vi "DeQueue State.vi"(8 "error in":errorcluster, 10 "Timeout (-1)":i32=-1, 11 "queue in":refnum<queue>) -> (0 "error out":errorcluster, 1 "Message Data":variant, 2 "Message":T1=enum."Load Data", 3 "queue out":refnum<queue>)   [LabVIEW 2020, in "Main_Process.lvlib" / "Internal Messaging Library.lvlib"]
doc: "Wait the indicated seconds or forever (-1) for the an element to enter the queue and then dequeue it and pass it out in the form of the message.\n\n2/2025 Erich Schlieper"
uses:
  Internal Messaging Library.lvlib
  Controls/Messaging Cluster.ctl
  Controls/Message.ctl
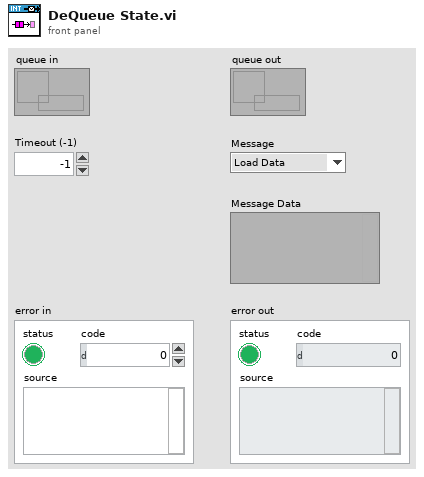
[diagram p1: front panel]
types:
  T1 = typedef "Main_Process.lvlib/Internal Messaging Library.lvlib/Message.ctl" = enum16{"Initialize", "Exit", "Error", "Load Data", "Add Project", "Edit Project", "Add Time Entry", "End Time Entry", "Save Project(s)", "Update Project List", "Update Task List", "Modify Time Entry", "Update Time Entry", "Delete Time Entry"}
  T2 = typedef "Main_Process.lvlib/Internal Messaging Library.lvlib/Messaging Cluster.ctl" = cluster{"Message":T1, "Data":variant}
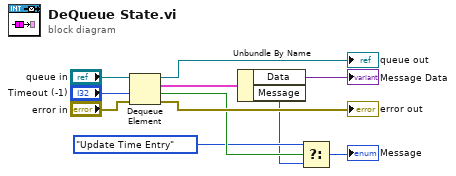
[diagram p0: block diagram]
diagram:
  n1 = Dequeue Element(queue="queue in", timeout in ms (-1)="Timeout (-1)", error in (no error)="error in") -> (queue out=→"queue out":refnum<queue>, element=w7:T2, timed out?=w4:bool, error out=→"error out":errorcluster)
  n2 = Unbundle By Name(w7) -> ("Data"=→"Message Data":variant, "Message"=w1:T1)
  n3 = Select(t=Message."Update Time Entry", s=w4, f=w1) -> (s? t:f=→"Message":T1)
